vi "ReadAndSaveData.vi"(0 "object in":refnum<class "MTEC_Async.lvclass">, 1 "tdms file":refnum<k34>, 2 "group name in (Untitled)":string, 5 "error in (no error)":errorcluster) -> (14 "object out":refnum<class "MTEC_Async.lvclass">, 16 "Latest Reading":T4 {"meTEC_CH2_Temperature Stability" items=["Temperature regulation is not active", "Is not stable", "Is stable"]; "meTEC_CH1_Device Status" items=["Initializing", "Ready", "Run", "Error", "Bootloader", "Reset in Progress"]; "meTEC_CH1_Temperature Stability" items=["Temperature regulation is not active", "Is not stable", "Is stable"]}, 17 "Buffer":T3(array[cluster]) {"DataOut"."meTEC_CH2_Temperature Stability" items=["Temperature regulation is not active", "Is not stable", "Is stable"]; "DataOut"."meTEC_CH1_Device Status" items=["Initializing", "Ready", "Run", "Error", "Bootloader", "Reset in Progress"]; "DataOut"."meTEC_CH1_Temperature Stability" items=["Temperature regulation is not active", "Is not stable", "Is stable"]}, 19 "error out":errorcluster)   [LabVIEW 2023, in "MTEC_Async.lvclass"]
uses:
  MTEC_Async.lvclass
  TEC LabVIEW Control Software v0.14/Source/LV Source/[meerstetter engineering TE Cooling]/TypeDefs/meTEC_ID 1200_Temperature is Stable.ctl
  TEC LabVIEW Control Software v0.14/Source/LV Source/[meerstetter engineering TE Cooling]/TypeDefs/meTEC_ID 104_Device Status.ctl
  MTEC_Async.lvclass/MTEC_Async.ctl
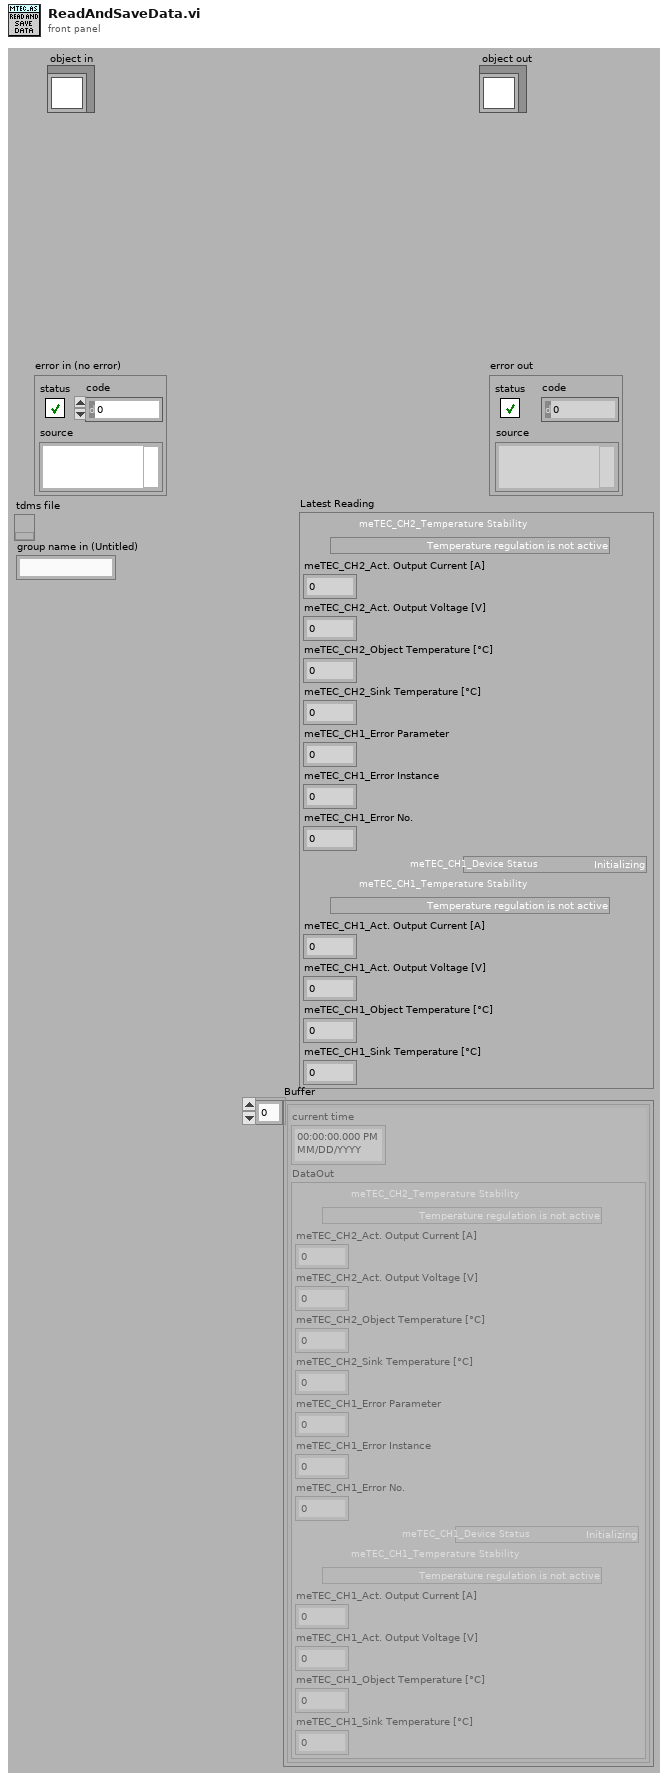
[diagram p1: front panel]
types:
  T1 = typedef "meTEC_ID 1200_Temperature is Stable.ctl" = i32
  T2 = typedef "meTEC_ID 104_Device Status.ctl" = i32
  T3 = cluster{"current time":timestamp, "DataOut":cluster{"meTEC_CH2_Temperature Stability":T1, "meTEC_CH2_Act. Output Current [A]":dbl, "meTEC_CH2_Act. Output Voltage [V]":dbl, "meTEC_CH2_Object Temperature [°C]":dbl, "meTEC_CH2_Sink Temperature [°C]":dbl, "meTEC_CH1_Error Parameter":i32, "meTEC_CH1_Error Instance":i32, "meTEC_CH1_Error No.":i32, "meTEC_CH1_Device Status":T2, "meTEC_CH1_Temperature Stability":T1, "meTEC_CH1_Act. Output Current [A]":dbl, "meTEC_CH1_Act. Output Voltage [V]":dbl, "meTEC_CH1_Object Temperature [°C]":dbl, "meTEC_CH1_Sink Temperature [°C]":dbl}}[]
  T4 = cluster{"meTEC_CH2_Temperature Stability":T1, "meTEC_CH2_Act. Output Current [A]":dbl, "meTEC_CH2_Act. Output Voltage [V]":dbl, "meTEC_CH2_Object Temperature [°C]":dbl, "meTEC_CH2_Sink Temperature [°C]":dbl, "meTEC_CH1_Error Parameter":i32, "meTEC_CH1_Error Instance":i32, "meTEC_CH1_Error No.":i32, "meTEC_CH1_Device Status":T2, "meTEC_CH1_Temperature Stability":T1, "meTEC_CH1_Act. Output Current [A]":dbl, "meTEC_CH1_Act. Output Voltage [V]":dbl, "meTEC_CH1_Object Temperature [°C]":dbl, "meTEC_CH1_Sink Temperature [°C]":dbl}
  T5 = cluster{"current time":timestamp, "DataOut":cluster{"meTEC_CH2_Temperature Stability":T1, "meTEC_CH2_Act. Output Current [A]":dbl, "meTEC_CH2_Act. Output Voltage [V]":dbl, "meTEC_CH2_Object Temperature [°C]":dbl, "meTEC_CH2_Sink Temperature [°C]":dbl, "meTEC_CH1_Error Parameter":i32, "meTEC_CH1_Error Instance":i32, "meTEC_CH1_Error No.":i32, "meTEC_CH1_Device Status":T2, "meTEC_CH1_Temperature Stability":T1, "meTEC_CH1_Act. Output Current [A]":dbl, "meTEC_CH1_Act. Output Voltage [V]":dbl, "meTEC_CH1_Object Temperature [°C]":dbl, "meTEC_CH1_Sink Temperature [°C]":dbl}}
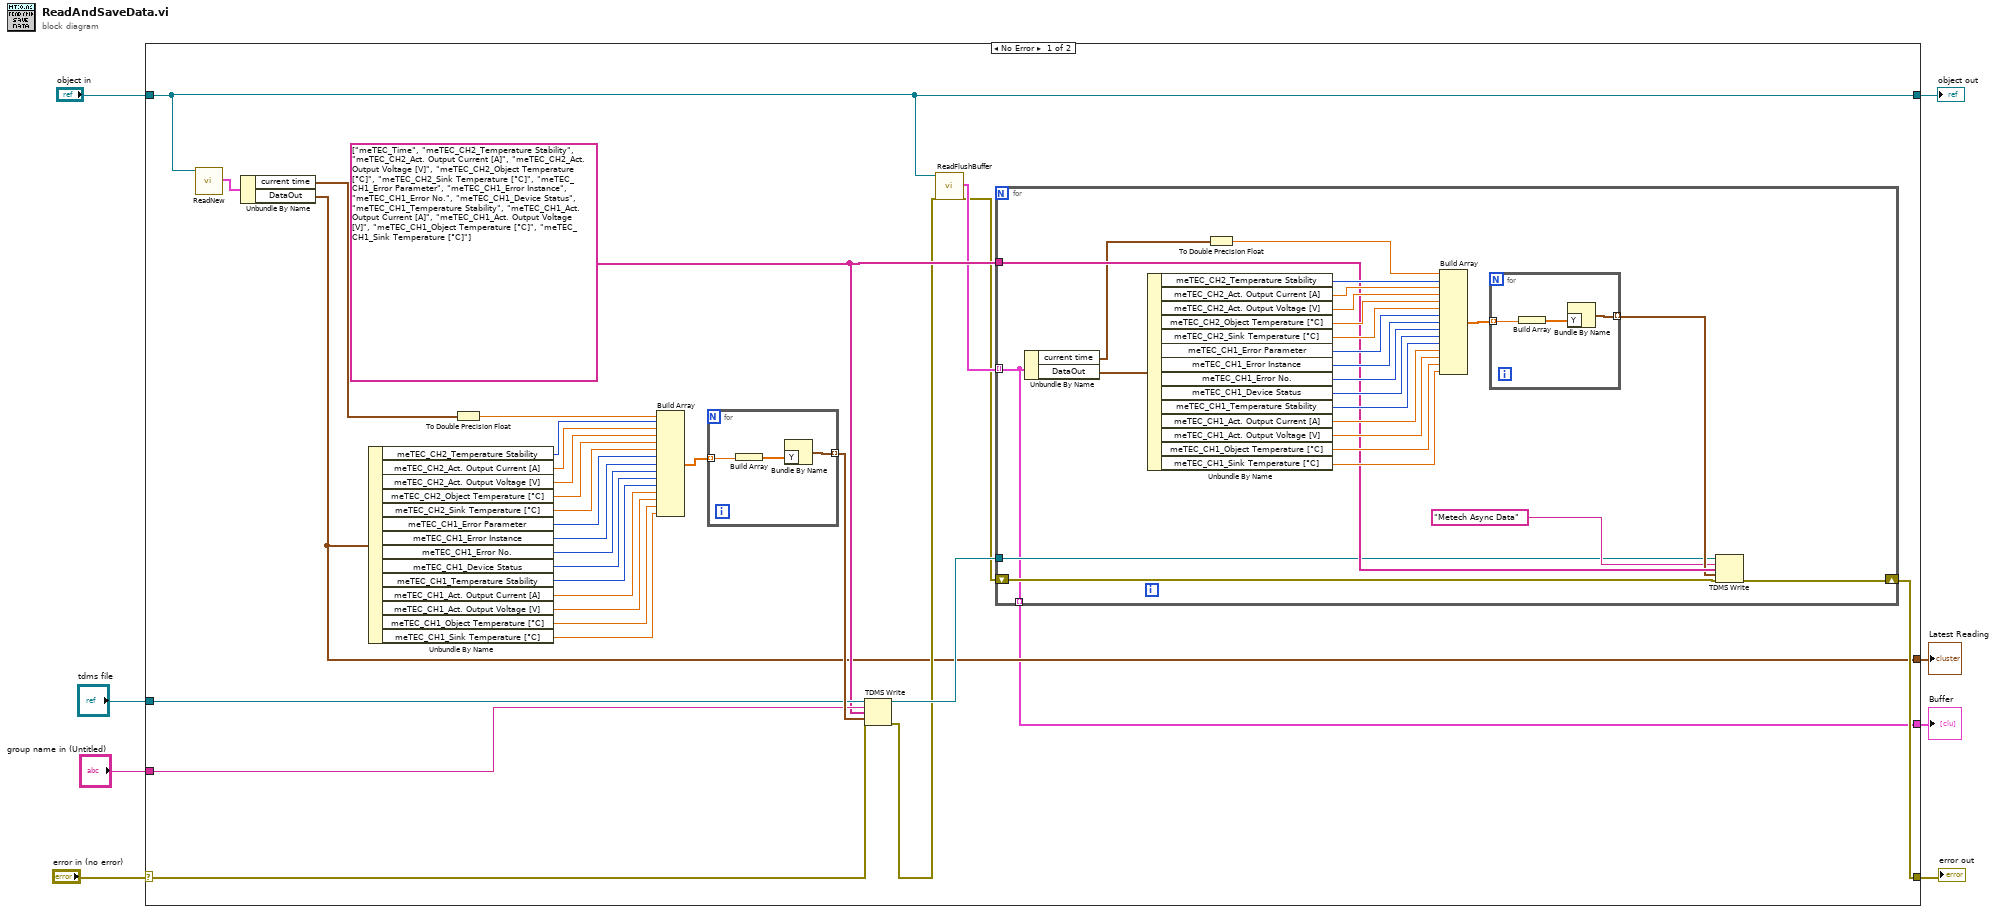
[diagram p0: block diagram]
diagram:
  n1 = case shown="No Error" "error in (no error)" {
    selector: "error in (no error)" -> [w20 w72]
    tunnel: [w13 w72] -> w7
    tunnel: [w19 w71] -> w5
    tunnel: "object in" -> [w19 w71]
    tunnel: "tdms file" -> [w22 _]
    tunnel: "group name in (Untitled)" -> [w21 _]
    tunnel: [w12 _] -> w2
    tunnel: [w9 _] -> w1
    frame No Error {
      w18 = string[] ["meTEC_Time", "meTEC_CH2_Temperature Stability", "meTEC_CH2_Act. Output Current [A]", "meTEC_CH2_Act. Output Voltage [V]", "meTEC_CH2_Object Temperature [°C]", "meTEC_CH2_Sink Temperature [°C]", "meTEC_CH1_Error Parameter", "meTEC_CH1_Error Instance", "meTEC_CH1_Error No.", "meTEC_CH1_Device Status", "meTEC_CH1_Temperature Stability", "meTEC_CH1_Act. Output Current [A]", "meTEC_CH1_Act. Output Voltage [V]", "meTEC_CH1_Object Temperature [°C]", "meTEC_CH1_Sink Temperature [°C]"] ("Array")
      n2 = call-dynamic "ReadNew.vi"("object in"=w19) -> ("notification"=w23:T5)  [unwired: 16 in, 2 out]
      n3 = Unbundle By Name(w23) -> ("current time"=w11:timestamp, "DataOut"=w12:T4)
      n4 = Unbundle By Name(w12) -> ("meTEC_CH2_Temperature Stability"=w39:T1, "meTEC_CH2_Act. Output Current [A]"=w38:dbl, "meTEC_CH2_Act. Output Voltage [V]"=w37:dbl, "meTEC_CH2_Object Temperature [°C]"=w36:dbl, "meTEC_CH2_Sink Temperature [°C]"=w35:dbl, "meTEC_CH1_Error Parameter"=w34:i32, "meTEC_CH1_Error Instance"=w33:i32, "meTEC_CH1_Error No."=w32:i32, "meTEC_CH1_Device Status"=w31:T2, "meTEC_CH1_Temperature Stability"=w30:T1, "meTEC_CH1_Act. Output Current [A]"=w29:dbl, "meTEC_CH1_Act. Output Voltage [V]"=w28:dbl, "meTEC_CH1_Object Temperature [°C]"=w27:dbl, "meTEC_CH1_Sink Temperature [°C]"=w26:dbl)
      n5 = To Double Precision Float(number=w11) -> (double precision float=w10:dbl)
      n6 = Build Array(w10, w39, w38, w37, w36, w35, w34, w33, w32, w31, w30, w29, w28, w27, w26) -> (w25:dbl[])
      n7 = for {
        tunnel: w25 -> [w70] mode=indexing
        tunnel: [w68] -> w24 mode=indexing
        n8 = Build Array(w70) -> (w69:dbl[])
        n9 = Bundle By Name("Y"=w69) -> (w68:waveform(dbl))  [unwired: 1 in]
      }
      n10 = TDMS Write(0:w22, 5:w21, 7:w18, 9:w24, 11:w20) -> (4:w16:refnum<k34>, 15:w14:errorcluster)  [unwired: 1 in, 2 out]
      n11 = call-dynamic "ReadFlushBuffer.vi"("object in"=w19, "error in (no error)"=w14) -> ("Stored Data"=w17:T3, "error out"=w15:errorcluster)  [unwired: 15 in, 1 out]
      n12 = for {
        tunnel: w18 -> [w49]
        tunnel: w17 -> [w40] mode=indexing
        tunnel: w16 -> [w45]
        tunnel: [w40] -> w9 mode=indexing
        shift-right: [w43] -> w13
        shift-left: w15 -> [w44]
        n13 = Unbundle By Name(w40) -> ("current time"=w42:timestamp, "DataOut"=w47:T4)
        n14 = Unbundle By Name(w47) -> ("meTEC_CH2_Temperature Stability"=w50:T1, "meTEC_CH2_Act. Output Current [A]"=w51:dbl, "meTEC_CH2_Act. Output Voltage [V]"=w52:dbl, "meTEC_CH2_Object Temperature [°C]"=w53:dbl, "meTEC_CH2_Sink Temperature [°C]"=w54:dbl, "meTEC_CH1_Error Parameter"=w55:i32, "meTEC_CH1_Error Instance"=w56:i32, "meTEC_CH1_Error No."=w57:i32, "meTEC_CH1_Device Status"=w58:T2, "meTEC_CH1_Temperature Stability"=w59:T1, "meTEC_CH1_Act. Output Current [A]"=w60:dbl, "meTEC_CH1_Act. Output Voltage [V]"=w61:dbl, "meTEC_CH1_Object Temperature [°C]"=w62:dbl, "meTEC_CH1_Sink Temperature [°C]"=w63:dbl)
        n15 = To Double Precision Float(number=w42) -> (double precision float=w41:dbl)
        n16 = Build Array(w41, w50, w51, w52, w53, w54, w55, w56, w57, w58, w59, w60, w61, w62, w63) -> (w64:dbl[])
        n17 = for {
          tunnel: w64 -> [w67] mode=indexing
          tunnel: [w65] -> w48 mode=indexing
          n18 = Build Array(w67) -> (w66:dbl[])
          n19 = Bundle By Name("Y"=w66) -> (w65:waveform(dbl))  [unwired: 1 in]
        }
        n20 = TDMS Write(0:w45, 5:"Metech Async Data" ("group name in (Untitled)"), 7:w49, 9:w48, 11:w44) -> (15:w43:errorcluster)  [unwired: 1 in, 3 out]
      }
    }
    frame Error {
    }
  }
  "error out" <- w7
  "object out" <- w5
  "Latest Reading" <- w2
  "Buffer" <- w1
